vi "Old Aging.vi"() -> ()   [LabVIEW 2023]
uses:
  <vilib>/Utility/file.llb/Read Delimited Spreadsheet (string).vi
  <vilib>/Utility/file.llb/Write Delimited Spreadsheet (string).vi
panel:
  out "Path":string
  out "Work_Order":string="XXXXXXXXXXX"
  in  "Number of Racks":i32
  out "System Info":string[][](array[string])
  out "Gatetime":string
  out "Unit_Number":string="XXXXXXXXXXX"
  out "System":string
  out "Frequency Address":i16=8
  in  "Serial Numbers":string[](array[string])
  out "All Data":string[][][](array[string])
  in  "System Status":string
  in  "Number of Units":i32[](array[numeric]) min=0 max=64 step=32
  # "Aging System 3"
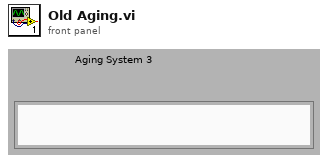
[diagram p1: front panel]
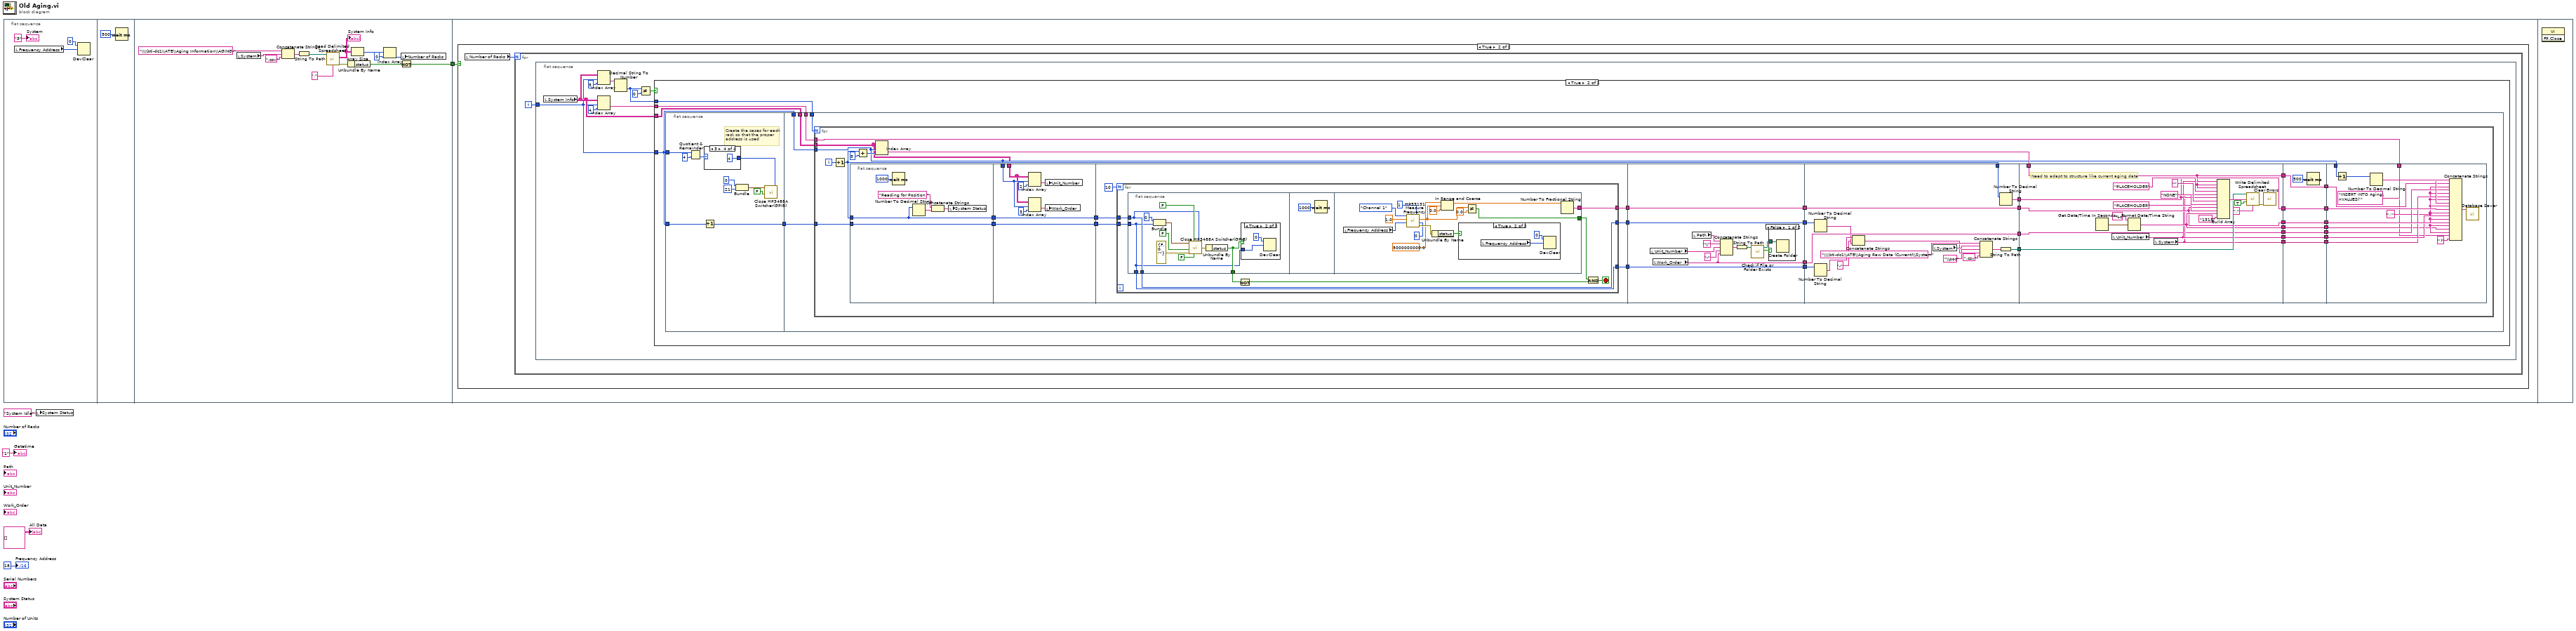
[diagram p0: block diagram]
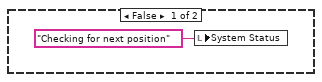
[diagram p3: hidden frame]
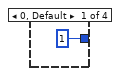
[diagram p4: hidden frame]
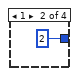
[diagram p5: hidden frame]
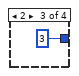
[diagram p6: hidden frame]
diagram:
  n1 = flat-sequence {
    tunnel: [w22] -> w1
    tunnel: w1 -> [w23]
    frame #0 {
      n2 = local read "Frequency Address"() -> (w7:i16)
      n3 = DevClear(3:w7, 4:0 ("GPIB Bus")) -> ()  [unwired: 1 in, 2 out]
      "System" <- "3" ("System")
    }
    frame #1 {
      n4 = Wait (ms)(milliseconds to wait=u32 500) -> ()  [unwired: 1 out]
    }
    frame #2 {
      n5 = local read "System"() -> (w19:string)
      n6 = Concatenate Strings("\\\\bti-dc1\\ATE\\Aging Information\\AGING-" ("string"), w19, ".csv" ("string")) -> (w18:string)
      n7 = String To Path(string=w18) -> (path=w13:path)
      n8 = call-poly <vilib>:"Read Delimited Spreadsheet.vi"("file path (dialog if empty)"=w13, "delimiter (\\t)"="," ("delimiter (\\t)")) -> ("all rows"=w12:string[][], "error out"=w11:errorcluster)  [unwired: 8 in, 4 out]
      "System Info" <- w12
      n9 = Unbundle By Name(w11) -> ("status"=w17:bool)
      n10 = Array Size(array=w12) -> (size(s)=w16:i32[])
      n11 = Index Array(array=w16, index=0) -> (element=w14:i32)
      n12 = Not(x=w17) -> (.not. x?=w22:bool)
      n13 = local write "Number of Racks"(w14) -> ()
    }
    frame #3 {
      n14 = case shown="True" w23 {
        frame False {
        }
        frame True {
          n15 = local read "Number of Racks"() -> (w24:i32)
          n16 = for {
            N: w24 -> [_]
            i -> [w25]
            n17 = flat-sequence {
              tunnel: w25 -> [w27]
              frame #0 {
                n18 = local read "System Info"() -> (w28:string[][])
                n19 = Index Array(array=w28, index (row)=w27, index (col)=5 ("disabled index (col)")) -> (element=w34:string)
                n20 = Index Array(array=w28, index (row)=w27, index (col)=4 ("disabled index (col)")) -> (element=w26:string)
                n21 = Decimal String To Number(string=w34) -> (number=w30:i32)  [unwired: 2 in, 1 out]
                n22 = Not Equal?(x=w30, y=0) -> (x != y?=w32:bool)
                n23 = case shown="True" w32 {
                  tunnel: w27 -> [_ w39]
                  tunnel: w28 -> [_ w40]
                  tunnel: w30 -> [_ w37]
                  tunnel: w26 -> [_ w36]
                  frame False {
                    n24 = local write "System Status"("Checking for next position" ("System Status")) -> ()
                  }
                  frame True {
                    n25 = flat-sequence {
                      tunnel: w39 -> [w46]
                      tunnel: w39 -> [w42]
                      tunnel: [w41] -> w38
                      tunnel: w39 -> [w59]
                      tunnel: w40 -> [w58]
                      tunnel: w38 -> [w57]
                      tunnel: w37 -> [w56]
                      tunnel: w36 -> [w55]
                      frame #0 {
                        # "Create the cases for each\nrack so that the proper\naddress is used"
                        n26 = Quotient & Remainder(x=w46, y=4) -> (floor(x/y)=w49:i32)  [unwired: 1 out]
                        n27 = Increment(x=w42) -> (x+1=w41:i32)
                        n28 = case shown="3" w49 {
                          tunnel: [1 ("y") 2 ("y") 3 ("y") 4 ("y")] -> w48
                          frame 0, Default {
                          }
                          frame 1 {
                          }
                          frame 2 {
                          }
                          frame 3 {
                          }
                        }
                        n29 = Bundle(0, 21) -> (w50:cluster{i32, i32})  [unwired: 1 in]
                        n30 = call "Close HP3488A Switcher(GPIB).vi"("Device In"=w50, "Use Card# 5"=FALSE, "Position Number"=w48) -> ()  [unwired: 5 in, 1 out]
                      }
                      frame #1 {
                        n31 = for {
                          N: w56 -> [_]
                          tunnel: w57 -> [w93]
                          tunnel: w59 -> [w82]
                          tunnel: w58 -> [w65]
                          tunnel: w55 -> [w64]
                          i -> [w97]
                          n32 = Increment(x=w97) -> (x+1=w91:i32)
                          n33 = flat-sequence {
                            tunnel: [w99] -> w88
                            tunnel: w91 -> [w99]
                            tunnel: w93 -> [w98]
                            tunnel: [w98] -> w86
                            tunnel: w88 -> [w111]
                            tunnel: [w111] -> w87
                            tunnel: w86 -> [w110]
                            tunnel: [w110] -> w85
                            tunnel: w65 -> [w105]
                            tunnel: w82 -> [w106]
                            tunnel: [w117] -> w84
                            tunnel: w87 -> [w116]
                            tunnel: w85 -> [w114]
                            tunnel: [w113] -> w62
                            tunnel: [w112] -> w60
                            tunnel: w84 -> [w167]
                            tunnel: [w167] -> w83
                            tunnel: [w158] -> w80
                            tunnel: [w157] -> w63
                            tunnel: w62 -> [w157]
                            tunnel: [w156] -> w61
                            tunnel: w60 -> [w156]
                            tunnel: [w184] -> w96
                            tunnel: [w181] -> w95
                            tunnel: [w180] -> w94
                            tunnel: w91 -> [w182]
                            tunnel: w83 -> [w184]
                            tunnel: [w178] -> w81
                            tunnel: w80 -> [w178]
                            tunnel: w63 -> [w169]
                            tunnel: w61 -> [w170]
                            tunnel: w96 -> [w191]
                            tunnel: w89 -> [w186]
                            tunnel: w95 -> [w189]
                            tunnel: w94 -> [w197]
                            tunnel: [w192] -> w79
                            tunnel: [w191] -> w77
                            tunnel: [w190] -> w75
                            tunnel: [w189] -> w73
                            tunnel: [w188] -> w71
                            tunnel: [w187] -> w69
                            tunnel: w81 -> [w187]
                            tunnel: [w186] -> w67
                            tunnel: w79 -> [w211]
                            tunnel: [w211] -> w78
                            tunnel: w77 -> [w210]
                            tunnel: [w210] -> w76
                            tunnel: w75 -> [w209]
                            tunnel: [w209] -> w74
                            tunnel: w73 -> [w208]
                            tunnel: [w208] -> w72
                            tunnel: w71 -> [w207]
                            tunnel: [w207] -> w70
                            tunnel: w69 -> [w206]
                            tunnel: [w206] -> w68
                            tunnel: w67 -> [w205]
                            tunnel: [w205] -> w66
                            tunnel: w78 -> [w215]
                            tunnel: w76 -> [w225]
                            tunnel: w74 -> [w224]
                            tunnel: w82 -> [w213]
                            tunnel: w72 -> [w223]
                            tunnel: w70 -> [w221]
                            tunnel: w68 -> [w220]
                            tunnel: w66 -> [w219]
                            tunnel: w64 -> [w214]
                            frame #0 {
                              n34 = Wait (ms)(milliseconds to wait=u32 1000) -> ()  [unwired: 1 out]
                              n35 = Number To Decimal String(number=w99) -> (decimal integer string=w101:string)  [unwired: 1 in]
                              n36 = Concatenate Strings("Reading for Position " ("System Status"), w101) -> (w100:string)
                              n37 = local write "System Status"(w100) -> ()
                            }
                            frame #1 {
                              n38 = Index Array(array=w105, index (row)=w106, index (col)=2) -> (element=w108:string)
                              n39 = Index Array(array=w105, index (row)=w106, index (col)=3) -> (element=w104:string)
                              n40 = local write "Unit_Number"(w108) -> ()
                              n41 = local write "Work_Order"(w104) -> ()
                            }
                            frame #2 {
                              n42 = for {
                                N: 10 -> [_]
                                tunnel: [w126] -> w117
                                tunnel: w116 -> [w125]
                                tunnel: w114 -> [w122]
                                tunnel: [w119] -> w113
                                tunnel: [w118] -> w112
                                stop <- w121 stop-if-true
                                n43 = flat-sequence {
                                tunnel: w125 -> [w128]
                                tunnel: [w129] -> w124
                                tunnel: w122 -> [w127]
                                tunnel: [w128] -> w119
                                tunnel: [w127] -> w118
                                tunnel: [w144] -> w126
                                tunnel: [w141] -> w123
                                frame #0 {
                                n44 = Bundle(0, w127) -> (w131:cluster{i32, i32})  [unwired: 1 in]
                                n45 = call "Close HP3488A Switcher(GPIB).vi"("Device In"=w131, "reset"=FALSE, "Use Card# 5"=FALSE, "ID query"=FALSE, "error in (no error)"=errorcluster {"status"=FALSE, "code"=0, "source"=""}, "Position Number"=w128) -> ("error out"=w130:errorcluster)  [unwired: 2 in]
                                n46 = Unbundle By Name(w130) -> ("status"=w129:bool)
                                n47 = case shown="True" w129 {
                                tunnel: w127 -> [_ w137]
                                frame False {
                                }
                                frame True {
                                n48 = DevClear(3:w137, 4:0 ("GPIB Bus")) -> ()  [unwired: 1 in, 2 out]
                                }
                                }
                                }
                                frame #1 {
                                n49 = Wait (ms)(milliseconds to wait=u32 1000) -> ()  [unwired: 1 out]
                                }
                                frame #2 {
                                n50 = local read "Frequency Address"() -> (w152:i16)
                                n51 = call "HP53131 Measure Frequency.vi"("GPIB Bus"=0, "Number of Readings"=1, "GPIB Address"=w152, "Gate Time"=1.0 ("number"), "Channel(1,2,3)"=enum16{"Channel 1", "Channel 2", "Channel 3"}."Channel 1") -> ("error out"=w150:errorcluster, "Frequency"=w142:dbl)  [unwired: 1 in]
                                n52 = Unbundle By Name(w150) -> ("status"=w149:bool)
                                n53 = In Range and Coerce(upper limit=5000000000.0, x=w142, lower limit=0.0) -> (coerced(x)=w151:dbl)  [unwired: 1 out]
                                n54 = case shown="True" w149 {
                                frame False {
                                }
                                frame True {
                                n55 = local read "Frequency Address"() -> (w154:i16)
                                n56 = DevClear(3:w154, 4:0 ("GPIB Bus")) -> ()  [unwired: 1 in, 2 out]
                                }
                                }
                                n57 = Not Equal?(x=w142, y=0.0) -> (x != y?=w141:bool)
                                n58 = Number To Fractional String(number=w151) -> (F-format string=w144:string)  [unwired: 3 in]
                                }
                                }
                                n59 = Not(x=w124) -> (.not. x?=w120:bool)
                                n60 = And(x=w123, y=w120) -> (x .and. y?=w121:bool)
                              }
                            }
                            frame #3 {
                              n61 = local read "Unit_Number"() -> (w161:string)
                              n62 = local read "Work_Order"() -> (w158:string)
                              n63 = local read "Path"() -> (w163:string)
                              n64 = Concatenate Strings(w163, "\\" ("string"), w161, "-" ("string"), w158) -> (w159:string)
                              n65 = String To Path(string=w159) -> (path=w166:path)
                              n66 = call <vilib>:"Check if File or Folder Exists.vi"("path"=w166) -> ("file or folder exists?"=w165:bool, "dup path"=w164:path)  [unwired: 8 in, 1 out]
                              n67 = case shown="False" w165 {
                                tunnel: w164 -> [w168 _]
                                frame False {
                                n68 = Create Folder(path (use dialog)=w168) -> ()  [unwired: 2 in, 3 out]
                                }
                                frame True {
                                }
                              }
                            }
                            frame #4 {
                              n69 = Number To Decimal String(number=w169) -> (decimal integer string=w174:string)  [unwired: 1 in]
                              n70 = Number To Decimal String(number=w170) -> (decimal integer string=w175:string)  [unwired: 1 in]
                              n71 = Concatenate Strings(w175, "-" ("string"), w174) -> (w172:string)
                              n72 = local read "System"() -> (w176:string)
                              n73 = Concatenate Strings("\\\\bti-dc1\\ATE\\Aging Raw Data (Current)\\System" ("string"), w176, "\\pos" ("string"), w172, ".csv" ("string")) -> (w183:string)
                              n74 = String To Path(string=w183) -> (path=w180:path)
                              n75 = Number To Decimal String(number=w182) -> (decimal integer string=w181:string)  [unwired: 1 in]
                            }
                            frame #5 {
                              # "Need to adapt to structure like current aging data"
                              n76 = Get Date/Time In Seconds() -> (seconds since 1Jan1904=w203:timestamp)
                              n77 = local read "Unit_Number"() -> (w190:string)
                              n78 = Format Date/Time String(time format string (%c)="%c", seconds (now)=w203) -> (date/time string=w192:string)  [unwired: 1 in]
                              n79 = local read "System"() -> (w188:string)
                              n80 = Build Array(w190, w186, w186, "PLACEHOLDER" ("element"), w188, w189, "" ("element"), "NONE" ("element"), w191, "PLACEHOLDER" ("element"), w192, "1313" ("element")) -> (w199:string[])
                              n81 = call-poly <vilib>:"Write Delimited Spreadsheet.vi"("file path (dialog if empty)"=w197, "1D data"=w199, "append to file? (new file:F)"=TRUE, "delimiter (\\t)"="," ("delimiter (\\t)")) -> ("error out"=w185:errorcluster)  [unwired: 10 in, 1 out]
                              n82 = call <vilib>:"Clear Errors.vi"("error in (no error)"=w185) -> ()  [unwired: 5 in, 2 out]
                            }
                            frame #6 {
                              n83 = Wait (ms)(milliseconds to wait=u32 500) -> ()  [unwired: 1 out]
                            }
                            frame #7 {
                              w217 = "','" ("string")
                              n84 = Increment(x=w213) -> (x+1=w212:i32)
                              n85 = Number To Decimal String(number=w212) -> (decimal integer string=w222:string)  [unwired: 1 in]
                              n86 = Concatenate Strings("INSERT INTO Aging\nVALUES('" ("SQL Query"), w219, w217, w220, w217, w221, w217, w222, w217, w223, w217, w224, w217, w225, w217, w215, w217, w214, "')" ("string")) -> (w218:string)
                              n87 = call "Database Saver.vi"("Command"=w218) -> ()  [unwired: 11 in]
                            }
                          }
                          n88 = Add(x=w91, y=5) -> (x+y=w90:i32)
                          n89 = Index Array(array=w65, index (row)=w82, index (col)=w90) -> (element=w89:string)
                        }
                      }
                    }
                  }
                }
              }
            }
          }
        }
      }
    }
    frame #4 {
      n90 = invoke class="VI" method="FP.Close"() -> ()  [unwired: 3 in, 3 out]
    }
  }
  n91 = local write "System Status"("System Idle" ("System Status")) -> ()
  "All Data" <- string[][][] [] ("All Data")
  "Frequency Address" <- i16 18 ("Frequency Address")
  "Gatetime" <- "1" ("Gatetime")
